vi "selectMonitor.vi"() -> (3 "monitor to use":i32)   [LabVIEW 2017]
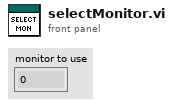
[diagram p1: front panel]
types:
  T1 = typedef "LVAllMonitorsDisplayTypeDef.ctl" = cluster{"Bounds":cluster{"Left":i16, "Top":i16, "Right":i16, "Bottom":i16}, "Depth":i16}[]
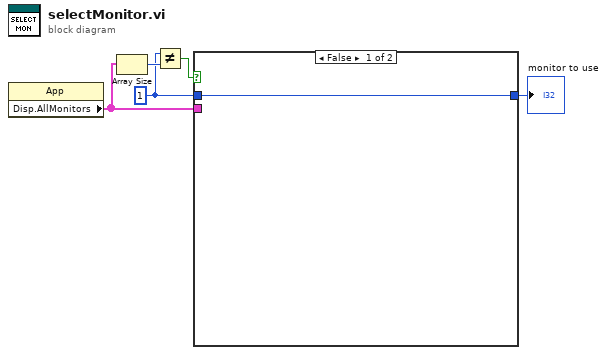
[diagram p0: block diagram]
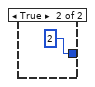
[diagram p2: hidden frame]
diagram:
  w3 = 1 ("x")
  n1 = property class="App"() -> ("Disp.AllMonitors"=w2:T1)  [unwired: 2 in, 2 out]
  n2 = Array Size(array=w2) -> (size(s)=w5:i32)
  n3 = Not Equal?(x=w3, y=w5) -> (x != y?=w4:bool)
  n4 = case shown="False" w4 {
    tunnel: [w6 u16 2 ("Front Panel Window:Monitor")] -> w1
    tunnel: w3 -> [w6 _]
    tunnel: w2 -> [_ _]
    frame False {
    }
    frame True {
    }
  }
  "monitor to use" <- w1
